vi "Read session ref.vi"(11 "CCD in":refnum<class "CCD.lvclass">) -> (2 "session ref":refnum<vi>, 3 "CCD out":refnum<class "CCD.lvclass">)   [LabVIEW 2016, in "Hardware.lvlib" / "CCD.lvlib" / "CCD.lvclass"]
uses:
  <userlib>/Common Components/Hardware/CCD/CCD/CCD.lvclass
  <vilib>/userdefined/High Color/IMAQdx.ctl
  <userlib>/Common Components/Hardware/CCD/CCD/CCD.lvclass/CCD.ctl
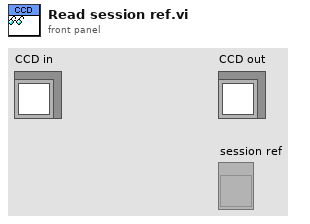
[diagram p1: front panel]
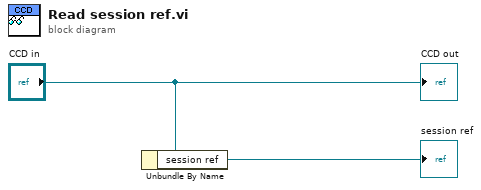
[diagram p0: block diagram]
diagram:
  n1 = Unbundle By Name("CCD in") -> ("session ref"=→"session ref":refnum<vi>)
  "CCD out" <- "CCD in"
